vi "PCO_Convert16TOCOL16.vi"(0 "ph":u64, 1 "height":i32, 2 "swap_colors":bool, 5 "mode":i32, 7 "icolmode":i32, 9 "width":i32, 11 "error in (no error)":errorcluster {"code" format="%x"}, 12 "raw_image(U16)":u16[][](array[numeric])=array1x4097[4097 elements]) -> (4 "ph out":u64, 6 "ErrorMessage":i32 format="%x", 8 "image (U64)":T1(array[cluster]), 15 "error out":errorcluster {"code" format="%x"})   [LabVIEW 2019, in "Convert.lvlib"]
doc: "int PCOCONVERT_API PCO_Convert16TOCOL16(HANDLE ph, int mode, int icolmode, int width, int height, word *b16in, word *b16out);"
uses:
  Convert.lvlib
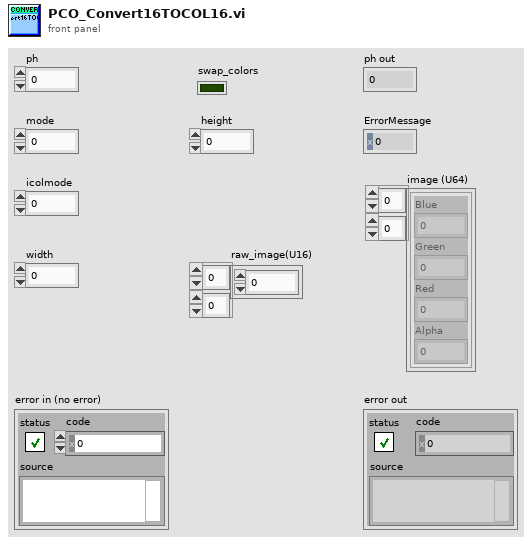
[diagram p1: front panel]
types:
  T1 = cluster{"Blue":u16, "Green":u16, "Red":u16, "Alpha":u16}[][]
  T2 = cluster{"Plane 4 (alpha)":u16, "Plane 1 (Red)":u16, "Plane 2 (Green)":u16, "Plane 3 (Blue)":u16}
  T3 = cluster{"Blue":u16, "Green":u16, "Red":u16, "Alpha":u16}
  T4 = cluster{"Plane 4 (alpha)":u16, "Plane 1 (Red)":u16, "Plane 2 (Green)":u16, "Plane 3 (Blue)":u16}[]
  T5 = cluster{"Plane 4 (alpha)":u16, "Plane 1 (Red)":u16, "Plane 2 (Green)":u16, "Plane 3 (Blue)":u16}[][]
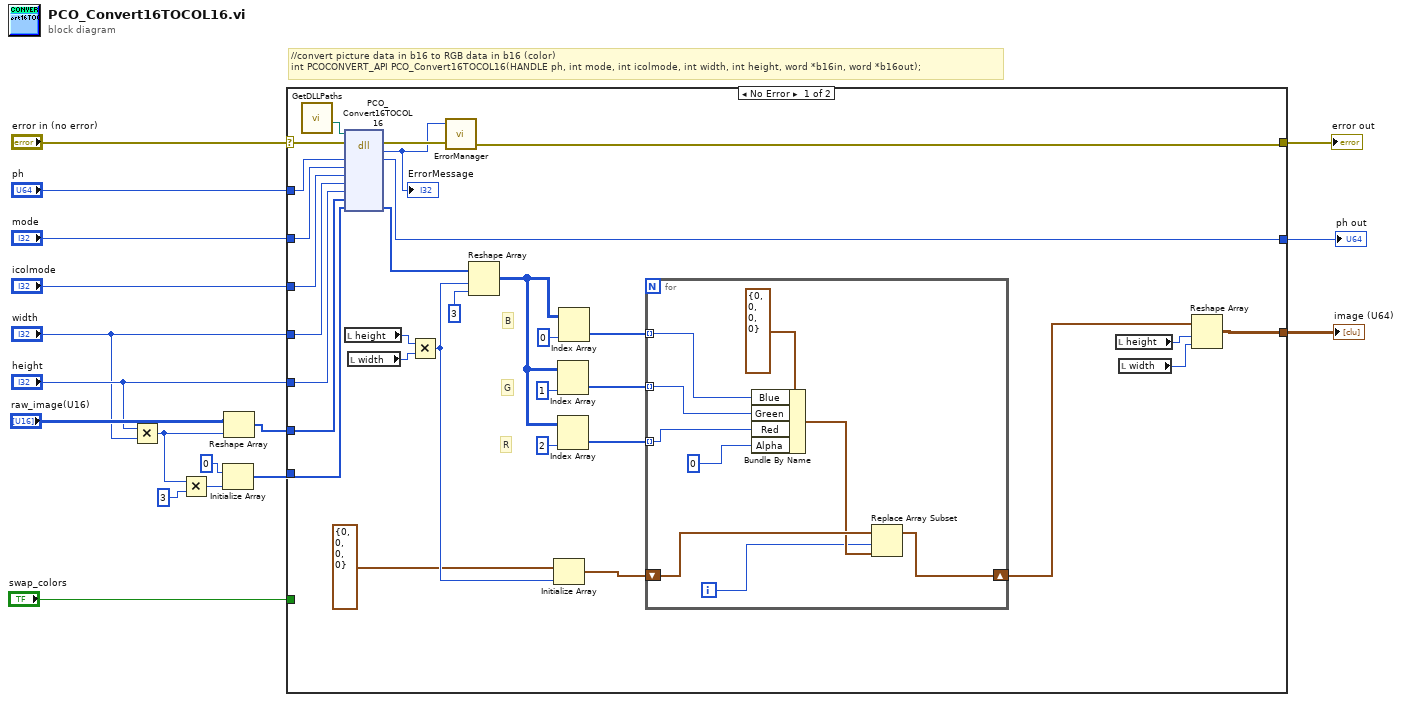
[diagram p0: block diagram]
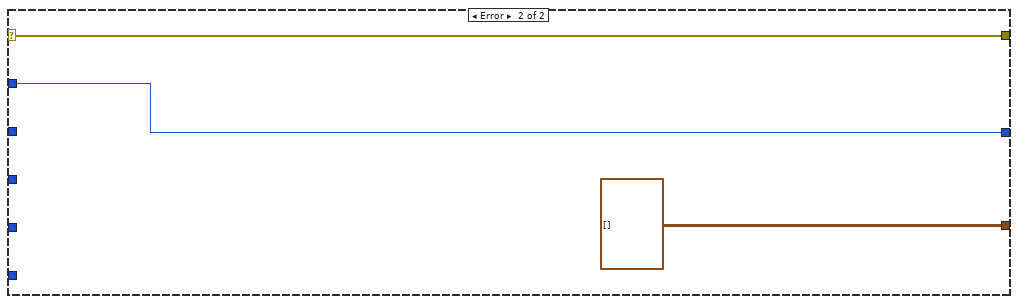
[diagram p2: hidden frame]
diagram:
  # "//convert picture data in b16 to RGB data in b16 (color)\nint PCOCONVERT_API PCO_Convert16TOCOL16(HANDLE ph, int mode, int icolmode, int width, int height, word *b16in, word *b16out);"
  n1 = Multiply(x="height", y="width") -> (x*y=w4:i32)
  n2 = Multiply(x=w4, y=3) -> (x*y=w5:i32)
  n3 = Initialize Array(u16 0 ("element"), w5) -> (w13:u16[])
  n4 = Reshape Array("raw_image(U16)", w4) -> (w8:u16[])
  n5 = case shown="No Error" "error in (no error)" {
    selector: "error in (no error)" -> [w40 w60]
    tunnel: "ph" -> [w48 w59]
    tunnel: [w47 w59] -> w16
    tunnel: "mode" -> [w46 _]
    tunnel: "icolmode" -> [w45 _]
    tunnel: w8 -> [w44 _]
    tunnel: w13 -> [w43 _]
    tunnel: [w38 w60] -> w11
    tunnel: "height" -> [w42 _]
    tunnel: "width" -> [w41 _]
    tunnel: [w22 T1 []] -> w1
    tunnel: "swap_colors" -> [_ _]
    frame No Error {
      # "R"
      # "G"
      # "B"
      n6 = call "GetDLLPaths.vi"() -> ("PCO_Conv_Path"=w36:path)  [unwired: 8 in, 3 out]
      n7 = dll-call lib="?" fn="PCO_Convert16TOCOL16"(path in=w36, error in=w40, "ph"=w48, "mode"=w46, "icolmode"=w45, "width"=w41, "height"=w42, "b16in"=w44, "b16out"=w43) -> (error out=w39:errorcluster, "return type"=w37:i32, "ph"=w47:u64, "b16out"=w35:u16[])  [unwired: 6 in, 1 out]
      "ErrorMessage" <- w37
      n8 = local read "height"() -> (w34:i32)
      n9 = local read "width"() -> (w33:i32)
      n10 = Multiply(x=w34, y=w33) -> (x*y=w23:i32)
      n11 = call "ErrorManager.vi"("error in (no error)"=w39, "error code"=w37) -> ("error out"=w38:errorcluster)  [unwired: 2 in, 1 out]
      n12 = Reshape Array(w35, w23, 3 ("dimension size")) -> (w28:u16[][])
      n13 = Initialize Array(T2 {"Plane 4 (alpha)"=0, "Plane 1 (Red)"=0, "Plane 2 (Green)"=0, "Plane 3 (Blue)"=0}, w23) -> (w24:T4)
      n14 = Index Array(array=w28, index (col)=1 ("disabled index (col)")) -> (element=w26:u16[])  [unwired: 1 in]
      n15 = Index Array(array=w28, index (col)=2 ("disabled index (col)")) -> (element=w25:u16[])  [unwired: 1 in]
      n16 = Index Array(array=w28, index (col)=0 ("disabled index (col)")) -> (element=w27:u16[])  [unwired: 1 in]
      n17 = for {
        tunnel: w27 -> [w54] mode=indexing
        tunnel: w26 -> [w55] mode=indexing
        tunnel: w25 -> [w56] mode=indexing
        shift-right: [w50] -> w21
        shift-left: w24 -> [w53]
        i -> [w51]
        n18 = Bundle By Name(cluster=T3 {"Blue"=0, "Green"=0, "Red"=0, "Alpha"=0}, "Blue"=w54, "Green"=w55, "Red"=w56, "Alpha"=u16 0 ("element")) -> (w52:T3)
        n19 = Replace Array Subset(array=w53, new element=w52, index=w51) -> (w50:T4)
      }
      n20 = local read "height"() -> (w20:i32)
      n21 = local read "width"() -> (w19:i32)
      n22 = Reshape Array(w21, w20, w19) -> (w22:T5)
    }
    frame Error {
    }
  }
  "ph out" <- w16
  "error out" <- w11
  "image (U64)" <- w1
